vi "GlobalExp.vi"() -> ()   [LabVIEW 2019, in "Global.lvlib"]
uses:
  Global.lvlib
  MasterExpControl.ctl
panel:
  in  "GlobalExp":T1={"Main Steps"=0.0, "Main Runs"=0.0, "ExpStatus"=enum."Stop", "Main Current Step"=0.0, "ExpNum"=0.0, "NewData"=FALSE, "date"="", "command"="", "Stop"=FALSE, "Pause"=FALSE, "Mathematica"="", "Main/Meta"=FALSE, "UpdateMath"=FALSE, "Camera"=FALSE, "MetaExpOver"=FALSE, "NextMetaExp"=FALSE}
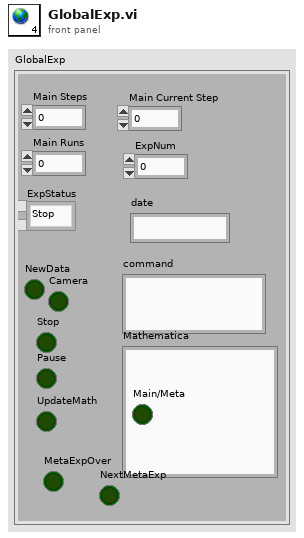
[diagram p1: front panel]
types:
  T1 = typedef "MasterExpControl.ctl" = cluster{"Main Steps":dbl, "Main Runs":dbl, "ExpStatus":enum16{"Innit", "Stop", "Idle", "MainRunning", "AuxRunning"}, "Main Current Step":dbl, "ExpNum":dbl, "NewData":bool, "date":string, "command":string, "Stop":bool, "Pause":bool, "Mathematica":string, "Main/Meta":bool, "UpdateMath":bool, "Camera":bool, "MetaExpOver":bool, "NextMetaExp":bool}
diagram:
